vi "Measure.vi"(8 "error in":errorcluster, 10 "Measure Type":u16(ring) items=["Voltage", "Current", "Power"], 11 "VISA resource name":refnum<visa-resource-name>) -> (0 "error out":errorcluster, 2 "Measurement":dbl, 3 "VISA resource name out":refnum<visa-resource-name>)   [LabVIEW 2015, in "IT6700H.lvlib"]
doc: "The command is used to measure and return the current voltage/current/power output value through the detection resistor inside the power supply.\n<b>Measure Type</b>\n0: Voltage\n1: Current\n2: Power"
uses:
  <instrlib>/IT6700H/IT6700H.lvlib
panel:
  in  "Max Timeout(ms)":u32=10000
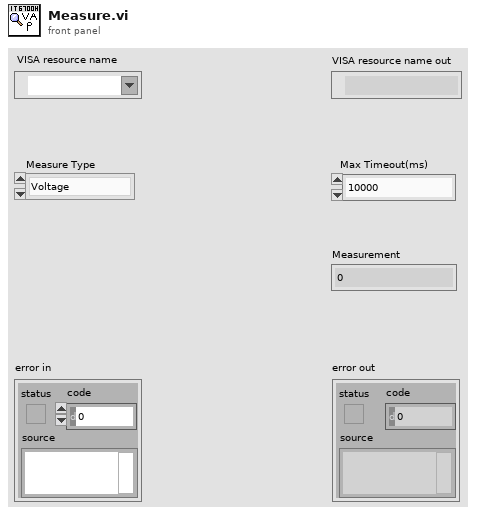
[diagram p1: front panel]
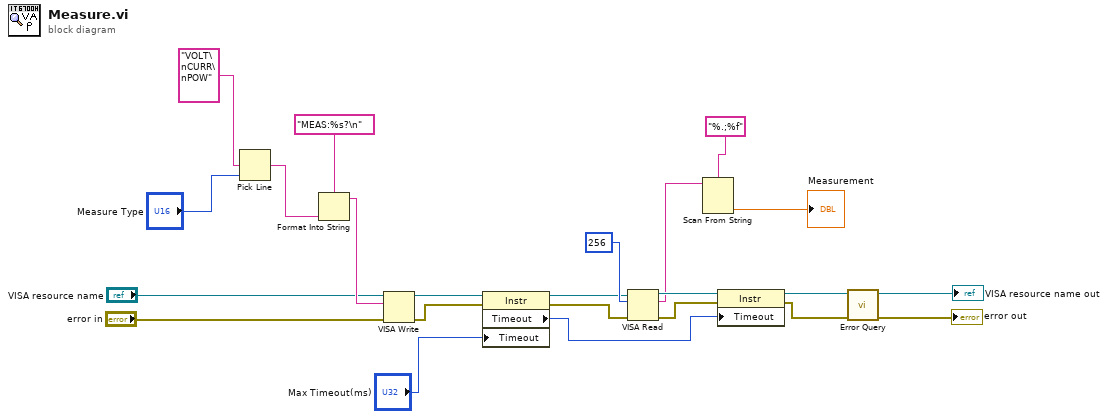
[diagram p0: block diagram]
diagram:
  n1 = Pick Line(multi-line string="VOLT\nCURR\nPOW", line index="Measure Type") -> (output string=w21:string)  [unwired: 1 in]
  n2 = Format Into String(format string="MEAS:%s?\n", w21) -> (resulting string=w19:string)  [unwired: 2 in, 1 out]
  n3 = VISA Write(VISA resource name="VISA resource name", write buffer=w19, error in (no error)="error in") -> (VISA resource name out=w13:refnum<visa-resource-name>, error out=w11:errorcluster)  [unwired: 1 out]
  n4 = property class="Instr"(reference=w13, error in=w11, "Timeout"="Max Timeout(ms)") -> (reference out=w12:refnum<visa-resource-name>, error out=w10:errorcluster, "Timeout"=w6:u32)
  n5 = VISA Read(VISA resource name=w12, byte count=256, error in (no error)=w10) -> (VISA resource name out=w7:refnum<visa-resource-name>, read buffer=w3:string, error out=w5:errorcluster)  [unwired: 1 out]
  n6 = Scan From String(format string="%.;%f", input string=w3) -> (output 1=→"Measurement":dbl)  [unwired: 3 in, 3 out]
  n7 = property class="Instr"(reference=w7, error in=w5, "Timeout"=w6) -> (reference out=w8:refnum<visa-resource-name>, error out=w4:errorcluster)
  n8 = call <instrlib>:"Error Query.vi"("error in"=w4, "VISA resource name"=w8) -> ("error out"=→"error out":errorcluster, "VISA resource name out"=→"VISA resource name out":refnum<visa-resource-name>)  [unwired: 6 in, 2 out]
